vi "LED0.vi"(11 "LED0":bool) -> ()   [LabVIEW 2021]
uses:
  <vilib>/rvi/eio/common/nirviEmuTemplateMethod_errors.vi
  <vilib>/eio/EIONode/EIONode.xnode
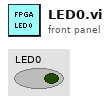
[diagram p1: front panel]
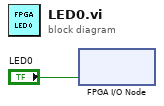
[diagram p0: block diagram]
diagram:
  n1 = xnode "FPGA I/O Node"("LED0"="LED0") -> ()  [unwired: 1 in, 1 out]
